vi "Main_complete.vi"() -> ()   [LabVIEW 2015]
uses:
  <vilib>/myRIO/Instrument Drivers/Onboard IO/I2C/typedefs/I2C User Configuration.ctl
  <vilib>/myRIO/Instrument Drivers/Onboard IO/I2C/typedefs/I2C Transfer Rate.ctl
  <vilib>/Platform/TimedLoop/XDataNode/timing_clust.ctl
  <vilib>/Platform/TimedLoop/XDataNode/nitl_modes.ctl
  <vilib>/Platform/TimedLoop/XDataNode/wakeup.ctl
  <vilib>/myRIO/Instrument Drivers/Onboard Devices/Accelerometer/typedefs/Accelerometer Reference.ctl
  <vilib>/myRIO/Common/Instrument Driver Framework/Utilities/typedefs/myRIO Generic Hardware Reference.ctl
  <vilib>/myRIO/Common/Instrument Driver Framework/Utilities/typedefs/Hardware Version Enum.ctl
  <vilib>/myRIO/Common/Instrument Driver Framework/Utilities/typedefs/myRIO v1.0 Reference.ctl
  <vilib>/myRIO/Common/Instrument Driver Framework/Utilities/typedefs/Generic FPGA Reference.ctl
  <vilib>/myRIO/Common/Instrument Driver Framework/myRIO v1.0/Accelerometer/typedefs/Accelerometer Channels List.ctl
  <vilib>/myRIO/Common/Instrument Driver Framework/myRIO v1.0/Accelerometer/typedefs/Accelerometer Channels Enum.ctl
  <vilib>/userdefined/High Color/nirio_resource_hc.ctl
  <vilib>/myRIO/Common/Instrument Driver Framework/myRIO v1.0/Encoder/typedefs/Encoder Signal Mode.ctl
  <vilib>/myRIO/Instrument Drivers/Onboard IO/Encoder/typedefs/Encoder Reference.ctl
  <vilib>/myRIO/Common/Instrument Driver Framework/myRIO v1.0/Encoder/typedefs/Encoder Channels Enum.ctl
  <vilib>/myRIO/Common/Instrument Driver Framework/myRIO v1.0/Encoder/typedefs/Encoder Configuration v1.0.ctl
  <vilib>/myRIO/Instrument Drivers/Onboard IO/PWM/typedefs/PWM Reference.ctl
  <vilib>/myRIO/Common/Instrument Driver Framework/myRIO v1.0/PWM/typedefs/PWM Channels Enum.ctl
  <vilib>/myRIO/Instrument Drivers/Onboard IO/PWM/typedefs/PWM Configuration.ctl
  <vilib>/myRIO/Instrument Drivers/Onboard IO/DIO/typedefs/DIO Reference.ctl
  <vilib>/myRIO/Common/Instrument Driver Framework/myRIO v1.0/DIO/typedefs/DIO Channels List.ctl
  <vilib>/myRIO/Common/Instrument Driver Framework/myRIO v1.0/DIO/typedefs/DIO Channels Enum.ctl
  <vilib>/myRIO/Common/Instrument Driver Framework/Utilities/vis/Is FPGA Ref Available.vi
  <vilib>/myRIO/Common/Instrument Driver Framework/myRIO v1.0/Encoder/vis/myRIO v1.1 Open Encoder.vi
  <vilib>/myRIO/Common/Instrument Driver Framework/myRIO v1.0/PWM/vis/myRIO v1.1 Open PWM.vi
  <vilib>/myRIO/Instrument Drivers/Onboard IO/PWM/vis/Set Duty Cycle and Frequency.vi
  <vilib>/myRIO/Common/Instrument Driver Framework/myRIO v1.0/DIO/vis/myRIO v1.1 Open DIO.vi
  <vilib>/myRIO/Common/Instrument Driver Framework/myRIO v1.0/Accelerometer/vis/myRIO v1.1 Open Accelerometer.vi
  <vilib>/myRIO/Common/Instrument Driver Framework/myRIO v1.0/I2C/vis/myRIO v1.1 Open I2C.vi
  <vilib>/myRIO/Common/Instrument Driver Framework/Utilities/vis/Validate Channels.vi
  <vilib>/myRIO/Common/Instrument Driver Framework/myRIO v1.0/Encoder/vis/myRIO v1.0 Reserve Encoder.vi
  <vilib>/myRIO/Common/Instrument Driver Framework/myRIO v1.0/PWM/vis/myRIO v1.0 Reserve PWM.vi
  <vilib>/myRIO/Common/Instrument Driver Framework/myRIO v1.0/DIO/vis/myRIO v1.0 Reserve DIO.vi
  <vilib>/myRIO/Common/Instrument Driver Framework/myRIO v1.0/Accelerometer/vis/myRIO v1.0 Reserve Accelerometer.vi
  <vilib>/myRIO/Common/Instrument Driver Framework/myRIO v1.0/UART/vis/myRIO v1.0 Close UART.vi
  <vilib>/myRIO/Common/Instrument Driver Framework/myRIO v1.0/I2C/vis/myRIO v1.0 Reserve I2C.vi
  <vilib>/myRIO/Common/Instrument Driver Framework/myRIO v1.0/Encoder/vis/myRIO v1.0 Build MUX Configuration Encoder.vi
  <vilib>/myRIO/Common/Instrument Driver Framework/myRIO v1.0/Resource Manager/vis/myRIO v1.0 Reserve Channel List.vi
  <vilib>/myRIO/Common/Instrument Driver Framework/myRIO v1.0/PWM/vis/myRIO v1.0 Build MUX Configuration PWM.vi
  <vilib>/myRIO/Common/Instrument Driver Framework/myRIO v1.0/DIO/vis/myRIO v1.0 Build MUX Configuration DIO.vi
  <vilib>/myRIO/Common/Instrument Driver Framework/myRIO v1.0/Accelerometer/vis/myRIO v1.0 Build MUX Configuration Accelerometer.vi
  <vilib>/myRIO/Common/Instrument Driver Framework/myRIO v1.0/I2C/vis/myRIO v1.0 Build MUX Configuration I2C.vi
  <vilib>/myRIO/Common/Instrument Driver Framework/myRIO v1.0/Resource Manager/vis/myRIO v1.0 Create Configuration List.vi
  <vilib>/myRIO/Common/Instrument Driver Framework/myRIO v1.0/Resource Manager/vis/myRIO v1.0 Reserve Channel.vi
  <vilib>/myRIO/Common/Instrument Driver Framework/myRIO v1.0/Resource Manager/vis/myRIO v1.0 Unreserve Channel.vi
  <vilib>/myRIO/Common/Instrument Driver Framework/myRIO v1.0/Resource Manager/vis/myRIO v1.0 Build Mutex Name.vi
  <vilib>/Utility/VariantDataType/GetNumericInfo.vi
  <vilib>/Utility/error.llb/Error Cluster From Error Code.vi
  <vilib>/myRIO/Common/Instrument Driver Framework/myRIO v1.0/myRIO v1.1 Open.vi
  <vilib>/myRIO/Common/Instrument Driver Framework/Utilities/vis/IO Manager.vi
  <vilib>/myRIO/Common/Instrument Driver Framework/Utilities/vis/Configuration Manager.vi
  <vilib>/myRIO/Common/Instrument Driver Framework/myRIO v1.0/Resource Manager/vis/myRIO v1.0 Configure IO.vi
  <vilib>/myRIO/Common/Instrument Driver Framework/myRIO v1.0/myRIO v1.0 Close.vi
  <vilib>/myRIO/Common/Instrument Driver Framework/myRIO v1.0/I2C/vis/myRIO v1.0 Configure I2C.vi
  <vilib>/myRIO/Common/Instrument Driver Framework/myRIO v1.0/I2C/vis/myRIO v1.0 Write I2C.vi
  <vilib>/myRIO/Common/Instrument Driver Framework/myRIO v1.0/Accelerometer/vis/myRIO v1.0 Get Scaling Constant Accelerometer.vi
  <vilib>/myRIO/Common/Instrument Driver Framework/myRIO v1.0/Accelerometer/vis/myRIO v1.0 Read Accelerometer.vi
  <vilib>/myRIO/Common/Instrument Driver Framework/myRIO v1.0/Encoder/vis/myRIO v1.0 Configure Encoder.vi
  <vilib>/myRIO/Common/Instrument Driver Framework/myRIO v1.0/Encoder/vis/myRIO v1.0 Read Encoder.vi
  <vilib>/myRIO/Common/Instrument Driver Framework/myRIO v1.0/PWM/vis/myRIO v1.0 Write PWM.vi
  <vilib>/myRIO/Common/Instrument Driver Framework/myRIO v1.0/DIO/vis/myRIO v1.0 Write DIO.vi
  <vilib>/myRIO/Common/Instrument Driver Framework/myRIO v1.0/DIO/vis/myRIO v1.0 Read DIO.vi
  <vilib>/myRIO/Common/Instrument Driver Framework/myRIO v1.0/I2C/vis/myRIO v1.0 Read I2C.vi
  <vilib>/myRIO/Common/Instrument Driver Framework/Utilities/vis/FPGA Ref Manager.vi
  <vilib>/myRIO/Common/Instrument Driver Framework/myRIO v1.0/myRIO v1.0 Reset FPGA.vi
  <vilib>/myRIO/Common/Instrument Driver Framework/myRIO v1.0/IRQ/vis/myRIO v1.0 IRQ Info FGV.vi
  <vilib>/myRIO/Common/Instrument Driver Framework/myRIO v1.0/IRQ/vis/myRIO v1.0 Timer IRQ Info FGV.vi
  <vilib>/myRIO/Common/Instrument Driver Framework/myRIO v1.0/IRQ/vis/myRIO v1.0 ISR Agent.vi
  <vilib>/platform/TimedLoop/XDataNode/XDataNode.xnode
  <vilib>/myRIO/Express VI/Onboard Devices/Accelerometer/Accelerometer Express VI.xnode
  <vilib>/myRIO/Instrument Drivers/Onboard Devices/Accelerometer/vis/myRIO Accelerometer Open.xnode
  <vilib>/myRIO/Express VI/Onboard IO/Encoder/Encoder Express VI.xnode
  <vilib>/myRIO/Instrument Drivers/Onboard IO/Encoder/vis/myRIO Encoder Open.xnode
  <vilib>/myRIO/Express VI/Onboard IO/PWM/PWM Express VI.xnode
  <vilib>/myRIO/Instrument Drivers/Onboard IO/PWM/vis/myRIO PWM Open.xnode
  <vilib>/myRIO/Express VI/Onboard IO/DO/DO Express VI.xnode
  <vilib>/myRIO/Instrument Drivers/Onboard IO/DIO/vis/myRIO DIO Open.xnode
  <vilib>/myRIO/Instrument Drivers/Utilities/Utilities.lvlib
  <vilib>/myRIO/Instrument Drivers/Onboard IO/I2C/I2C.lvlib
  <vilib>/myRIO/Instrument Drivers/Onboard IO/DIO/DIO.lvlib
  <vilib>/Platform/TimedLoop/XDataNode/XDNodeRunTimeDep.lvlib
  <vilib>/ptbypt/NI_PtbyPt.lvlib
  <vilib>/myRIO/Instrument Drivers/Onboard Devices/Accelerometer/Accelerometer.lvlib
  <vilib>/myRIO/Instrument Drivers/Onboard IO/PWM/PWM.lvlib
  <vilib>/myRIO/Instrument Drivers/Onboard IO/Encoder/Encoder.lvlib
panel:
  in  "STOP":bool
  out "gyrodtheta_dps":dbl format="%0.2f"
  out "dtheta_wheel":dbl
  out "ang wheel vel":dbl(graph)
  out "theta_filter":dbl
  out "time":dbl
  out "theta_wheel_rad":dbl
  out "error out_motor":errorcluster
  in  "Reset Counter":bool
  out "Direction":bool
  in  "Enable":bool
  in  "PWM duty  [%]":dbl(slide) scale=-100.0..100.0
  in  "PWM freq [Hz]":dbl(slide)=100.0 scale=40.0..40000.0
  out "Z-Axis_accelrn":dbl
  out "dv":dbl
  out "Y-Axis Acceleration":dbl
  out "error out_gyro":errorcluster
  out "error out_acclr":errorcluster
  out "theta_deg":dbl format="%0.2f"
  in  "reset integrator":bool
  # "Gyroscope demo"
  # "DC MOTOR"
  # "ACCLEROMETER"
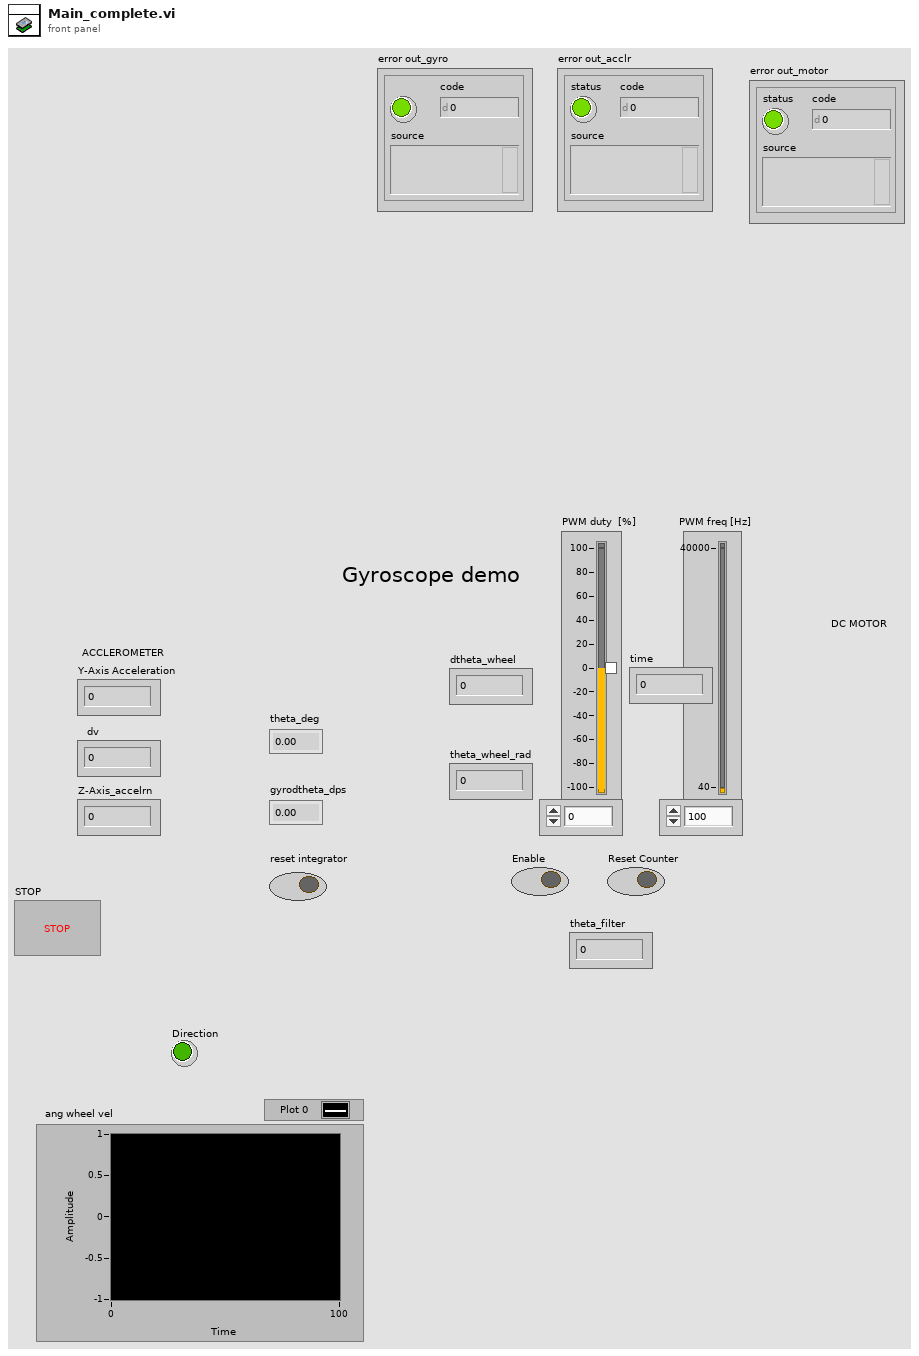
[diagram p1: front panel]
types:
  T1 = typedef "I2C.lvlib/I2C User Configuration.ctl" = cluster{"I2C Transfer Rate":T2}
  T2 = typedef "I2C.lvlib/I2C Transfer Rate.ctl" = enum16{"Standard mode (100 kbps)", "Fast mode (400 kbps)"}
  T3 = typedef "I2C.lvlib/I2C Reference.ctl" = cluster{"myRIO Reference":T4, "I2C Channels Enum":T8, "I2C Configuration":T9}
  T4 = typedef "myRIO Generic Hardware Reference.ctl" = cluster{"myRIO Model":T5, "myRIO Hardware Reference":T6}
  T5 = typedef "Hardware Version Enum.ctl" = enum16{"Unknown", "myRIO-1900", "myRIO-1950", "roboRIO"}
  T6 = typedef "myRIO v1.0 Reference.ctl" = cluster{"Generic FPGA Reference":T7, "Allow multiple opens":bool}
  T7 = typedef "Generic FPGA Reference.ctl" = refnum<k20>
  T8 = typedef "I2C Channels Enum.ctl" = enum16{"Not Connected", "A/I2C", "B/I2C", "I2C/I2C"}
  T9 = typedef "I2C.lvlib/I2C Configuration.ctl" = cluster{"I2C Transfer Rate":T2}
  T10 = typedef "DIO.lvlib/DIO Reference.ctl" = cluster{"myRIO Reference":T4, "DIO Channels List":T11}
  T11 = typedef "DIO Channels List.ctl" = T12[]
  T12 = typedef "DIO Channels Enum.ctl" = enum16{"Not Connected", "C/DIO0", "C/DIO1", "C/DIO2", "C/DIO3", "C/DIO4", "C/DIO5", "C/DIO6", "C/DIO7", "A/DIO0", "A/DIO1", "A/DIO2", "A/DIO3", "A/DIO4", "A/DIO5", "A/DIO6", "A/DIO7", "A/DIO8", "A/DIO9", "A/DIO10", "A/DIO11", "A/DIO12", "A/DIO13", "A/DIO14", "A/DIO15", "B/DIO0", "B/DIO1", "B/DIO2", "B/DIO3", "B/DIO4", "B/DIO5", "B/DIO6", "B/DIO7", "B/DIO8", "B/DIO9", "B/DIO10", "B/DIO11", "B/DIO12", "B/DIO13", "B/DIO14", "B/DIO15", "LED0", "LED1", "LED2", "LED3", "Button0", "DIO/DIO0", "DIO/DIO1", "DIO/DIO2", "DIO/DIO3", "DIO/DIO4", "DIO/DIO5", "DIO/DIO6", "DIO/DIO7", "DIO/DIO8", "DIO/DIO9", "SPI/CS0", "SPI/CS1", "SPI/CS2", "SPI/CS3", "LED RADIO (Green)", "LED RADIO (Red)", "LED COMM (Green)", "LED COMM (Red)", "LED MODE (Green)", "LED MODE (Red)"}
  T13 = typedef "XDNodeRunTimeDep.lvlib/timing_clust.ctl" = cluster{"Expected End [f-1]":u64, "Actual End [f-1]":u64, "Finished Late? [f-1]":bool, "Expected End [i-1]":u64, "Actual End [i-1]":u64, "Finished Late? [i-1]":bool, "Expected Start [i]":u64, "Actual Start [i]":u64, "Expected Start [f]":u64, "Actual Start [f]":u64, "Source Name":string, "Structure Name":string, "Period":i64, "Deadline":i64, "Offset":i64, "Start":i64, "Priority":i32, "Timeout":i32, "Mode":T14, "Wakeup Reason":T15, "Error":errorcluster, "Source Type":string, "Secondary Source Type":string, "Global End Time":u64, "Global Start Time":u64, "Frame Duration":u64, "Iteration Duration":u64, "Assigned CPU":i32, "I/O Scan Engine Mode":u32}
  T14 = typedef "XDNodeRunTimeDep.lvlib/nitl_modes.ctl" = enum32{"No Change", "Process missed periods, maintain original phase", "Discard missed periods, maintain original phase", "Process missed periods, ignore original phase", "Discard missed periods, ignore original phase"}
  T15 = typedef "XDNodeRunTimeDep.lvlib/wakeup.ctl" = enum32{"Normal", "Aborted", "Asynchronous wakeup", "Timing source error", "Timed loop error", "Timeout"}
  T16 = typedef "Encoder.lvlib/Encoder Reference.ctl" = cluster{"myRIO Reference":T4, "Encoder Channels Enum":T17}
  T17 = typedef "Encoder Channels Enum.ctl" = enum16{"Not Connected", "C/ENC0", "C/ENC1", "A/ENC", "B/ENC", "DIO/ENC0", "DIO/ENC1", "DIO/ENC2", "DIO/ENC3", "DIO/ENC4"}
  T18 = typedef "Encoder Signal Mode.ctl" = enum16{"Quadrature phase signal", "Step and direction signal"}
  T19 = typedef "nirio_resource_hc.ctl" = tag
  T20 = typedef "PWM.lvlib/PWM Reference.ctl" = cluster{"myRIO Reference":T4, "PWM Channels Enum":T21, "PWM Configuration":T22}
  T21 = typedef "PWM Channels Enum.ctl" = enum16{"Not Connected", "C/PWM0", "C/PWM1", "A/PWM0", "A/PWM1", "A/PWM2", "B/PWM0", "B/PWM1", "B/PWM2", "PWM/PWM0", "PWM/PWM1", "PWM/PWM2", "PWM/PWM3", "PWM/PWM4", "PWM/PWM5", "PWM/PWM6", "PWM/PWM7", "PWM/PWM8", "PWM/PWM9"}
  T22 = typedef "PWM.lvlib/PWM Configuration.ctl" = cluster{"Frequency":dbl, "Duty Cycle":dbl}
  T23 = typedef "Accelerometer.lvlib/Accelerometer Reference.ctl" = cluster{"myRIO Reference":T4, "Accelerometer Channels List":T24, "LSB Weight":dbl}
  T24 = typedef "Accelerometer Channels List.ctl" = T25[]
  T25 = typedef "Accelerometer Channels Enum.ctl" = enum16{"Not Connected", "X-Axis", "Y-Axis", "Z-Axis"}
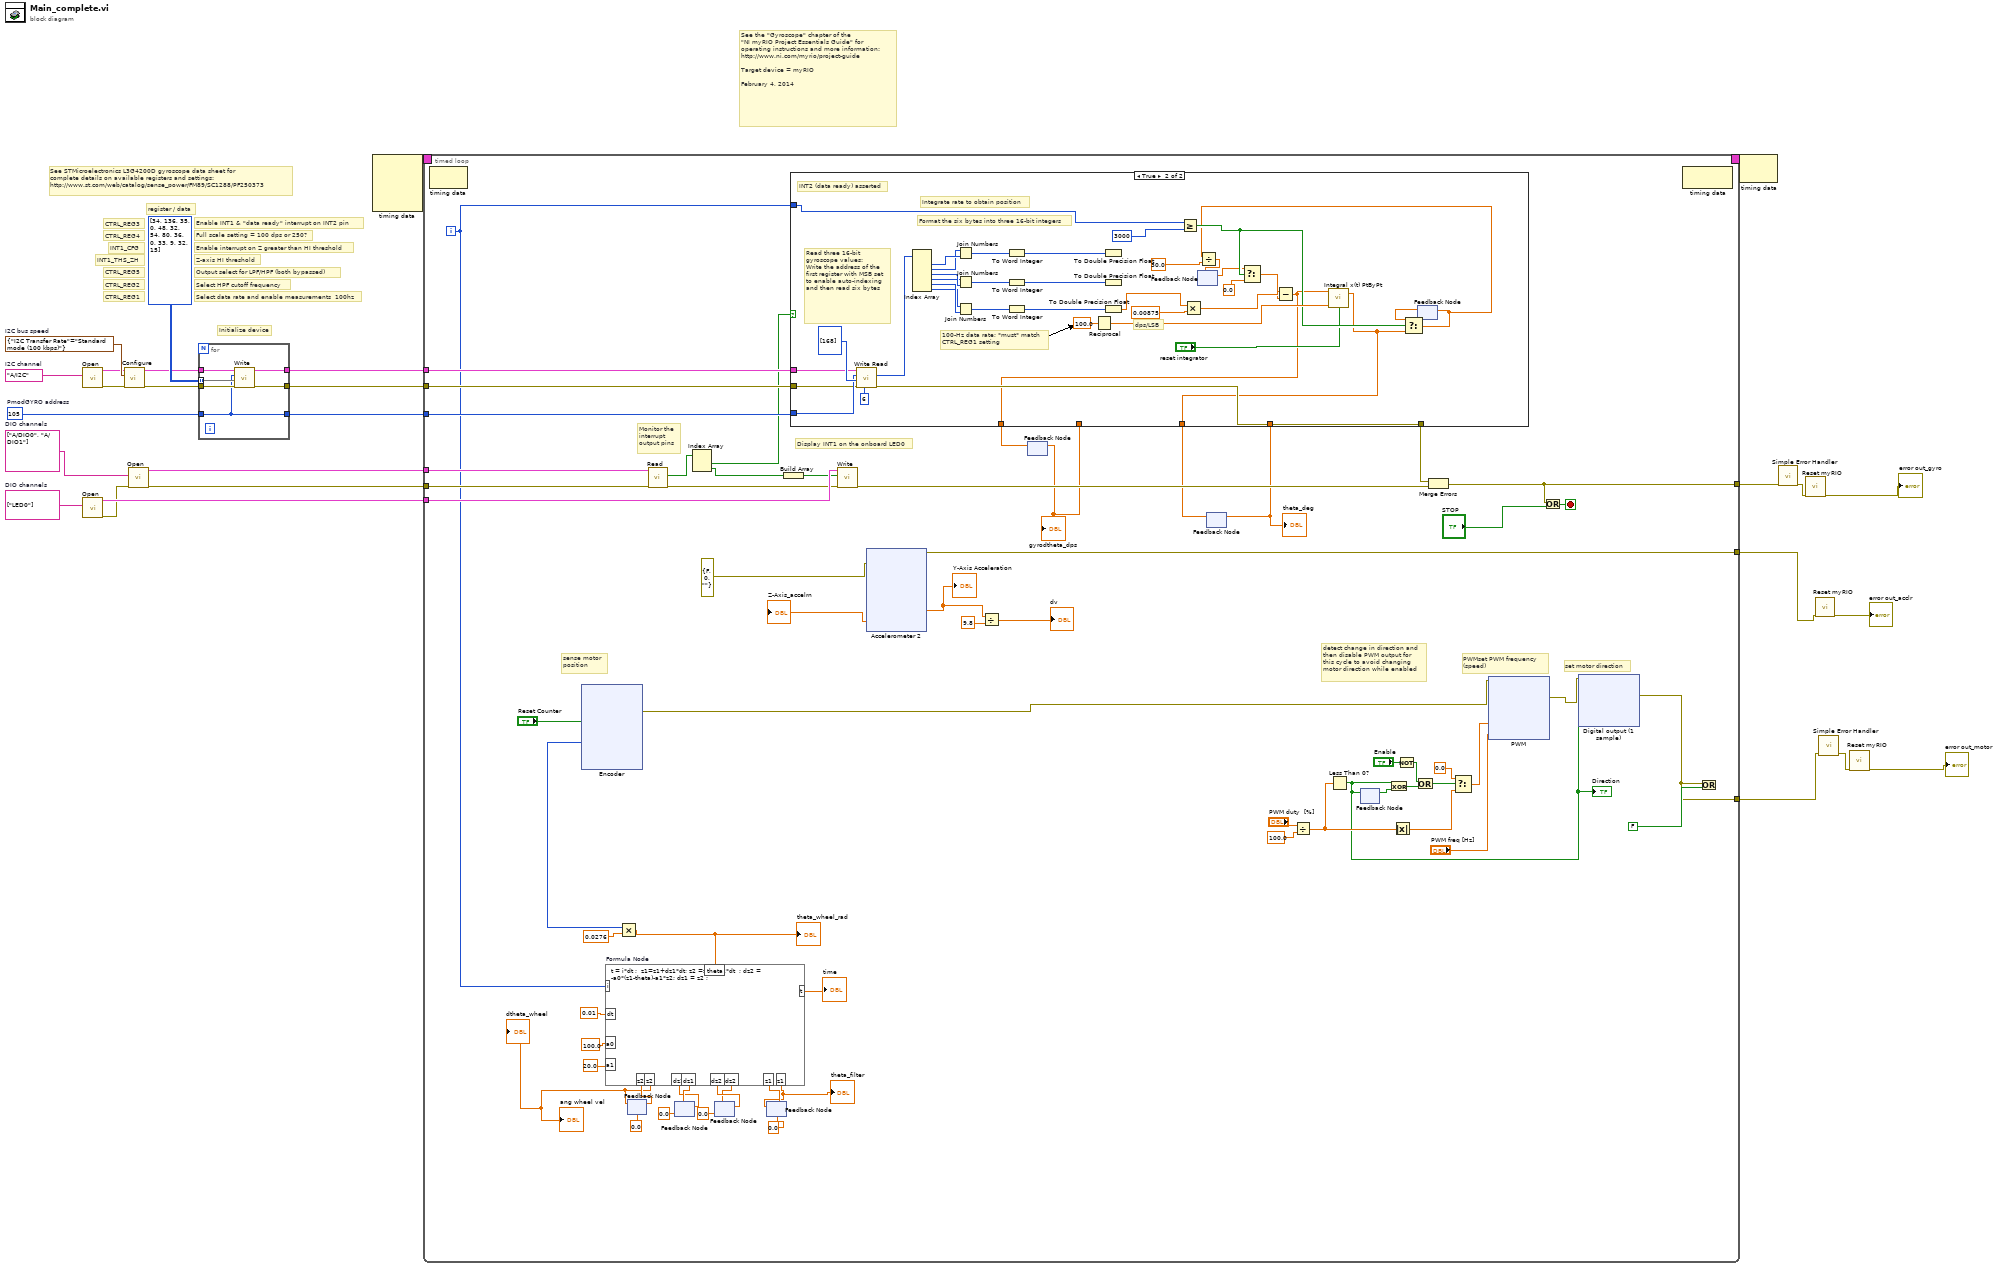
[diagram p0: block diagram]
diagram:
  w9 = tag[] ["LED0"]  # DIO channels
  w12 = tag[] ["A/DIO0", "A/DIO1"]  # DIO channels
  w24 = T1 {"I2C Transfer Rate"=enum."Standard mode (100 kbps)"}  # I2C bus speed
  w25 = tag "A/I2C"  # I2C channel
  w15 = u8 105  # PmodGYRO address
  # "See the \"Gyroscope\" chapter of the\n\"NI myRIO Project Essentials Guide\" for\noperating instructions and more information: \nhttp://www.ni.com/myrio/project-guide\n\nTarget device = myRIO\n\nFebruary 4, 2014"
  # "Enable INT1 & \"data ready\" interrupt on INT2 pin"
  # "CTRL_REG3"
  # "Select HPF cutoff frequency"
  # "CTRL_REG2"
  # "Output select for LPF/HPF (both bypassed)"
  # "CTRL_REG5"
  # "Initialize device"
  # "Select data rate and enable measurements  100hz"
  # "Z-axis HI threshold"
  # "Enable interrupt on Z greater than HI threshold"
  # "See STMicroelectronics L3G4200D gyroscope data sheet for\ncomplete details on available registers and settings:\nhttp://www.st.com/web/catalog/sense_power/FM89/SC1288/PF250373"
  # "CTRL_REG1"
  # "INT1_THS_ZH"
  # "INT1_CFG"
  # "Full scale setting = 100 dps or 250?"
  # "CTRL_REG4"
  # "register / data"
  n1 = call <vilib>:"Open.vi"("Channel Name"=w25) -> ("error out"=w22:errorcluster, "I2C Ref Out"=w23:T3)  [unwired: 9 in]
  n2 = call <vilib>:"Open.vi"("Channel Names"=w9) -> ("error out"=w7:errorcluster, "DIO Ref Out"=w8:T10)  [unwired: 9 in]
  n3 = call <vilib>:"Configure.vi"("error in (no error)"=w22, "I2C User Configuration"=w24, "I2C Ref In"=w23) -> ("error out"=w16:errorcluster, "I2C Ref Out"=w17:T3)  [unwired: 7 in]
  n4 = call <vilib>:"Open.vi"("error in (no error)"=w7, "Channel Names"=w12) -> ("error out"=w14:errorcluster, "DIO Ref Out"=w13:T10)  [unwired: 8 in]
  n5 = for {
    tunnel: [w33] -> w21
    tunnel: [w32] -> w20
    tunnel: [w28] -> w19
    tunnel: u8[][] [[34, 136], [35, 0], [48, 32], [54, 80], [36, 0], [33, 9], [32, 15]] ("Bytes to Write") -> [w31] mode=indexing
    tunnel: w17 -> [w30]
    tunnel: w16 -> [w29]
    tunnel: w15 -> [w28]
    n6 = call <vilib>:"Write.vi"("error in (no error)"=w29, "Bytes to Write"=w31, "Slave Address (7-bit)"=w28, "I2C Ref In"=w30) -> ("error out"=w33:errorcluster, "I2C Ref Out"=w32:T3)  [unwired: 6 in]
  }
  n7 = node-c288() -> (w11:T13)  [unwired: 4 in]
  n8 = timed-loop {
    tunnel: [w83] -> w26
    tunnel: w19 -> [w94]
    tunnel: w21 -> [w96]
    tunnel: w20 -> [w95]
    tunnel: w14 -> [w93]
    tunnel: w13 -> [w92]
    timing: w11 -> [_]
    timing-out: [_] -> w10
    tunnel: w8 -> [w88]
    tunnel: [w82] -> w5
    tunnel: [w59] -> w2
    i -> [w40]
    stop <- w97 stop-if-true
    # "sense motor \nposition"
    # "detect change in direction and\nthen disable PWM output for\nthis cycle to avoid changing\nmotor direction while enabled"
    # "PWMset PWM frequency\n(speed)"
    # "set motor direction"
    # "Display INT1 on the onboard LED0"
    # "Monitor the\ninterrupt\noutput pins"
    n9 = node-c288() -> ()  [unwired: 1 in, 1 out]
    n10 = xnode "Encoder"("Reset Counter"="Reset Counter") -> ("Counter Value"=w41:i32, "error out"=w73:errorcluster)  [unwired: 1 in, 2 out]
    n11 = Multiply(x=w41, y=0.0276) -> (x*y=w55:dbl)
    "theta_wheel_rad" <- w55
    n12 = feedback #1(0.0 ("input variable")) -> (w49:dbl)
    n13 = call <vilib>:"Read.vi"("error in (no error)"=w93, "DIO Ref In"=w92) -> ("error out"=w87:errorcluster, "Values"=w89:bool[])  [unwired: 7 in, 1 out]
    n14 = feedback #2(0.0 ("dz1")) -> (w47:dbl)
    n15 = Index Array "Index Array"(array=w89) -> (element #1=w90:bool, element #2=w85:bool)  [unwired: 2 in]
    n16 = feedback #3(0.0 ("dz2")) -> (w44:dbl)
    n17 = feedback #4(0.0 ("input variable")) -> (w52:dbl)
    n18 = formula code="t = i*dt ;  z1=z1+dz1*dt; z2 =z2+dz2*dt  ; dz2 = -a0*(z1-theta)-a1*z2; dz1 = z2 ;"("i"=w40, "dt"=0.01 ("y"), "theta"=w55, "a0"=100.0 ("input variable"), "a1"=20.0 ("input variable"), "z1"=w52, "z2"=w49, "dz1"=w47, "dz2"=w44) -> ("t"=→"time":dbl, "z1"=w43:dbl, "z2"=w39:dbl, "dz1"=w48:dbl, "dz2"=w42:dbl)
    "theta_filter" <- w43
    "ang wheel vel" <- w39
    "dtheta_wheel" <- w39
    n19 = feedback-in #1(w39) -> ()
    n20 = feedback-in #2(w48) -> ()
    n21 = feedback-in #3(w42) -> ()
    n22 = feedback-in #4(w43) -> ()
    n23 = Build Array "Build Array"(w85) -> (w86:bool[])
    n24 = call <vilib>:"Write.vi"("error in (no error)"=w87, "Values"=w86, "DIO Ref In"=w88) -> ("error out"=w84:errorcluster)  [unwired: 6 in, 1 out]
    n25 = xnode "Accelerometer 2"("error in (no error)"=errorcluster {"status"=FALSE, "code"=0, "source"=""}) -> ("Y-Axis"=w80:dbl, "Z-Axis"=→"Z-Axis_accelrn":dbl, "error out"=w82:errorcluster)  [unwired: 1 out]
    "Y-Axis Acceleration" <- w80
    n26 = Divide(x=w80, y=9.8) -> (x/y=→"dv":dbl)
    n27 = feedback #5() -> (w36:dbl)  [unwired: 1 in]
    "gyrodtheta_dps" <- w36
    n28 = feedback #6() -> (w34:dbl)  [unwired: 1 in]
    "theta_deg" <- w34
    n29 = case shown="True" w90 {
      tunnel: w96 -> [w257 w276]
      tunnel: w95 -> [_ w277]
      tunnel: w94 -> [_ w283]
      tunnel: [w257 w282] -> w91
      tunnel: w40 -> [_ w262]
      tunnel: [w255 w259] -> w35
      tunnel: [w256 w258] -> w37
      tunnel: w36 -> [w256 _]
      tunnel: w34 -> [w255 _]
      frame False {
        # "INT2 (data ready) deasserted"
      }
      frame True {
        # "dps/LSB"
        # "100-Hz data rate; *must* match\nCTRL_REG1 setting"
        # "Integrate rate to obtain position"
        # "INT2 (data ready) asserted"
        # "Read three 16-bit gyroscope values:\nWrite the address of the first register with MSB set to enable auto-indexing and then read six bytes"
        # "Format the six bytes into three 16-bit integers"
        n30 = call <vilib>:"Write Read.vi"("Byte Count"=u32 6, "error in (no error)"=w276, "Bytes to Write"=u8[] [168], "Slave Address (7-bit)"=w283, "I2C Ref In"=w277) -> ("error out"=w282:errorcluster, "Bytes Read"=w281:u8[])  [unwired: 3 in, 1 out]
        n31 = Index Array "Index Array"(array=w281) -> (element #1=w291:u8, element #2=w290:u8, element #3=w289:u8, element #4=w288:u8, element #5=w287:u8, element #6=w286:u8)  [unwired: 6 in]
        n32 = Join Numbers(hi=w290, lo=w291) -> ((hi.lo)=w294:u16)
        n33 = Join Numbers(hi=w288, lo=w289) -> ((hi.lo)=w293:u16)
        n34 = Join Numbers(hi=w286, lo=w287) -> ((hi.lo)=w292:u16)
        n35 = To Word Integer(number=w294) -> (16bit integer=w280:i16)
        n36 = To Word Integer(number=w293) -> (16bit integer=w279:i16)
        n37 = To Word Integer(number=w292) -> (16bit integer=w278:i16)
        n38 = Reciprocal(x=100.0 ("dt")) -> (1/x=w274:dbl)
        n39 = To Double Precision Float(number=w280) -> ()  [unwired: 1 out]
        n40 = To Double Precision Float(number=w279) -> ()  [unwired: 1 out]
        n41 = To Double Precision Float(number=w278) -> (double precision float=w272:dbl)
        n42 = Greater Or Equal?(x=w262, y=3000) -> (x >= y?=w270:bool)
        n43 = Multiply(x=w272, y=0.00875) -> (x*y=w265:dbl)
        n44 = feedback #7() -> (w266:dbl)  [unwired: 1 in]
        n45 = Select(t=w266, s=w270, f=0.0) -> (s? t:f=w264:dbl)
        n46 = Subtract(x=w265, y=w264) -> (x-y=w258:dbl)
        n47 = call <vilib>:"Integral x(t) PtByPt.vi"("initialize"="reset integrator", "dt"=w274, "x"=w258) -> ("integral x(t)"=w259:dbl)  [unwired: 1 in, 1 out]
        n48 = feedback #8() -> (w269:dbl)  [unwired: 1 in]
        n49 = Select(t=w269, s=w270, f=w259) -> (s? t:f=w260:dbl)
        n50 = Divide(x=w260, y=30.0 ("x")) -> (x/y=w267:dbl)
        n51 = feedback-in #7(w267) -> ()
        n52 = feedback-in #8(w260) -> ()
      }
    }
    n53 = feedback-in #5(w37) -> ()
    n54 = feedback-in #6(w35) -> ()
    n55 = Divide(x="PWM duty  [%]", y=100.0) -> (x/y=w63:dbl)
    n56 = Less Than 0?(x=w63) -> (x < 0?=w60:bool)
    "Direction" <- w60
    n57 = feedback #9() -> (w71:bool)  [unwired: 1 in]
    n58 = feedback-in #9(w60) -> ()
    n59 = Exclusive Or(1:w71, 2:w60) -> (0:w69:bool)
    n60 = Absolute Value(x=w63) -> (abs(x)=w61:dbl)
    n61 = Not(x="Enable") -> (.not. x?=w66:bool)
    n62 = Or(x=w66, y=w69) -> (x .or. y?=w68:bool)
    n63 = Merge Errors "Merge Errors"(w91, w84) -> (w83:errorcluster)
    n64 = Select(t=0.0 ("f"), s=w68, f=w61) -> (s? t:f=w62:dbl)
    n65 = xnode "PWM"("Duty Cycle"=w62, "Frequency [Hz]"="PWM freq [Hz]", "error in (no error)"=w73) -> ("error out"=w72:errorcluster)
    n66 = Or(x=w83, y="STOP") -> (x .or. y?=w97:bool)
    n67 = xnode "Digital output (1 sample)"("B/DIO0 (Pin 11)"=w60, "error in (no error)"=w72) -> ("error out"=w59:errorcluster)
    n68 = node-c288() -> ()  [unwired: 1 in, 1 out]
    n69 = Or(x=w59, y=FALSE ("[ESC]MOTOR")) -> ()  [unwired: 1 out]
  }
  n70 = node-c288(w10) -> ()  [unwired: 1 out]
  n71 = call <vilib>:"Simple Error Handler.vi"("error in (no error)"=w26) -> ("error out"=w27:errorcluster)  [unwired: 4 in, 4 out]
  n72 = call <vilib>:"Reset myRIO.vi"("error in (no error)"=w27) -> ("error out"=→"error out_gyro":errorcluster)  [unwired: 10 in]
  n73 = call <vilib>:"Reset myRIO.vi"("error in (no error)"=w5) -> ("error out"=→"error out_acclr":errorcluster)  [unwired: 10 in]
  n74 = call <vilib>:"Simple Error Handler.vi"("error in (no error)"=w2) -> ("error out"=w3:errorcluster)  [unwired: 4 in, 4 out]
  n75 = call <vilib>:"Reset myRIO.vi"("error in (no error)"=w3) -> ("error out"=→"error out_motor":errorcluster)  [unwired: 10 in]
